vi "Run Test Suite.vi"(8 "error in (no error)":errorcluster, 10 "Test Suite":refnum<class "LUnit Test Suite.lvclass">, 11 "Execution API In":refnum<class "Execution API.lvclass">) -> (0 "error out":errorcluster, 3 "Execution API Out":refnum<class "Execution API.lvclass">)   [LabVIEW 2020, in "Execution API.lvclass"]
doc: "Run all tests in a Test Suite."
uses:
  Execution API.lvclass
  C:/git/astemes-lunit/source/Framework/Result Observer/Result Observer.lvclass
  LUnit Test Suite.lvclass
  C:/git/astemes-lunit/source/Runnable.lvclass
  Execution API.lvclass/Execution API.ctl
  Framework/Test Runner/Test Runner.lvclass
  Framework/Plugin/Plugin.lvclass
  C:/git/astemes-lunit/source/User Interface/Execution API/Execution API.lvclass
  C:/git/astemes-lunit/source/LUnit Test Suite.lvclass
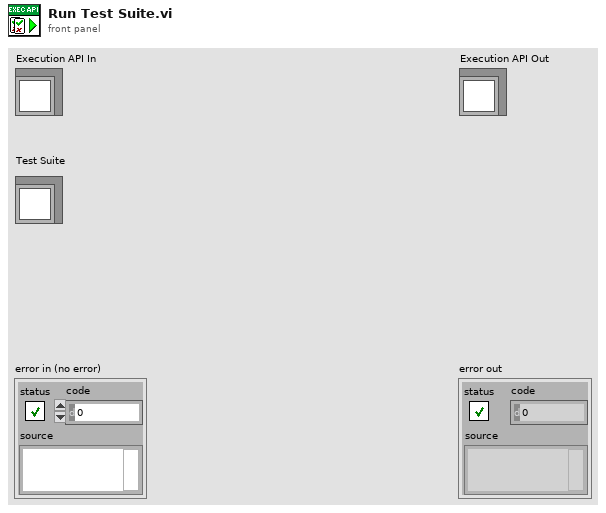
[diagram p1: front panel]
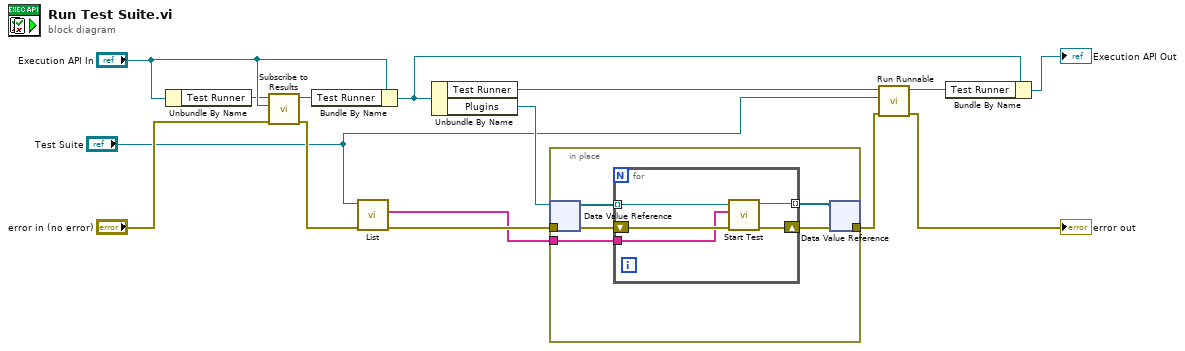
[diagram p0: block diagram]
diagram:
  n1 = Unbundle By Name("Execution API In") -> ("Test Runner"=w5:refnum<class "Test Runner.lvclass">)
  n2 = call-dynamic "Subscribe to Results.vi"("error in (no error)"="error in (no error)", "Result Observer"="Execution API In", "Test Runner In"=w5) -> ("error out"=w7:errorcluster, "Test Runner Out"=w6:refnum<class "Test Runner.lvclass">)  [unwired: 7 in]
  n3 = Bundle By Name(cluster="Execution API In", "Test Runner"=w6) -> (w9:refnum<class "Execution API.lvclass">)
  n4 = call "List.vi"("error in (no error)"=w7, "LUnit Test Suite In"="Test Suite") -> ("error out"=w3:errorcluster, "List of Runnables"=w2:string[])  [unwired: 8 in]
  n5 = Unbundle By Name(w9) -> ("Test Runner"=w15:refnum<class "Test Runner.lvclass">, "Plugins"=w4:refnum<data-value>)
  n6 = in-place {
    in-place-border: [w20] -> w11
    in-place-border: w3 -> [w19]
    in-place-border: w2 -> [w16]
    n7 = in-place-dvr #1(w4) -> (w18:refnum<class "Plugin.lvclass">[])  [unwired: 1 out]
    n8 = for {
      tunnel: w18 -> [w25] mode=indexing
      shift-right: [w24] -> w20
      shift-left: w19 -> [w23]
      tunnel: [w22] -> w17 mode=indexing
      tunnel: w16 -> [w21]
      n9 = call-dynamic "Start Test.vi"("error in (no error)"=w23, "Tests"=w21, "Plugin in"=w25) -> ("error out"=w24:errorcluster, "Plugin out"=w22:refnum<class "Plugin.lvclass">)  [unwired: 7 in]
    }
    n10 = in-place-dvr #1(w17) -> ()  [unwired: 2 out]
  }
  n11 = call-dynamic "Run Runnable.vi"("error in (no error)"=w11, "Runnable"="Test Suite", "Test Runner In"=w15) -> ("error out"=→"error out":errorcluster, "Test Runner Out"=w14:refnum<class "Test Runner.lvclass">)  [unwired: 7 in]
  n12 = Bundle By Name(cluster=w9, "Test Runner"=w14) -> (→"Execution API Out":refnum<class "Execution API.lvclass">)
